vi "readSHTJson.vi"(0 "JSON in":string, 3 "error in (no error)":errorcluster) -> (6 "error out":errorcluster, 7 "cluster":T1(array[cluster]), 8 "SHTListName":string[](array[string]), 9 "Temp2D":dbl[][](array[numeric]), 10 "RH2D":dbl[][](array[numeric]))   [LabVIEW 2018]
panel:
  out "Temp":dbl[](array[numeric])
  out "RH":dbl[](array[numeric])
  in  "Array in":T1(array[cluster])
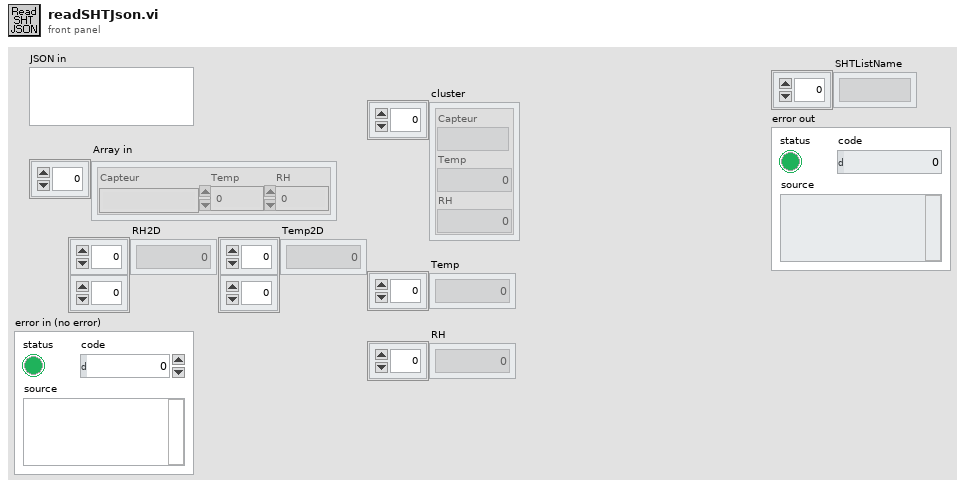
[diagram p1: front panel]
types:
  T1 = cluster{"Capteur":string, "Temp":dbl, "RH":dbl}[]
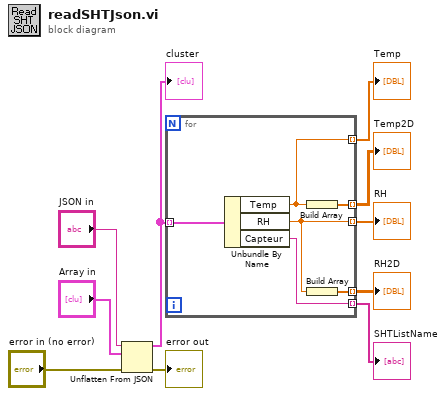
[diagram p0: block diagram]
diagram:
  n1 = Unflatten From JSON(JSON string="JSON in", type and defaults="Array in", error in (no error)="error in (no error)") -> (value=w7:T1, error out=→"error out":errorcluster)  [unwired: 4 in]
  "cluster" <- w7
  n2 = for {
    tunnel: w7 -> [w16] mode=indexing
    tunnel: [w14] -> w9 mode=indexing
    tunnel: [w15] -> w10 mode=indexing
    tunnel: [w13] -> w5 mode=indexing
    tunnel: [w12] -> w4 mode=indexing
    tunnel: [w11] -> w3 mode=indexing
    n3 = Unbundle By Name(w16) -> ("Temp"=w14:dbl, "RH"=w15:dbl, "Capteur"=w11:string)
    n4 = Build Array(w14) -> (w13:dbl[])
    n5 = Build Array(w15) -> (w12:dbl[])
  }
  "RH" <- w10
  "Temp" <- w9
  "Temp2D" <- w5
  "RH2D" <- w4
  "SHTListName" <- w3
